vi "mfTxTrchCoder.vi"(7 "coder_type":dbl, 8 "error in (no error)":errorcluster caption="错误输入（无错误）", 9 "input_num":dbl, 10 "pdch_data":dbl[](array[numeric]), 11 "Path":path) -> (0 "error out":errorcluster caption="错误输出", 3 "out_data":dbl[](array[numeric]))   [LabVIEW 2015]
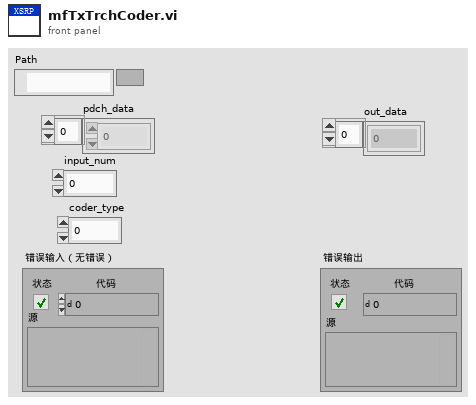
[diagram p1: front panel]
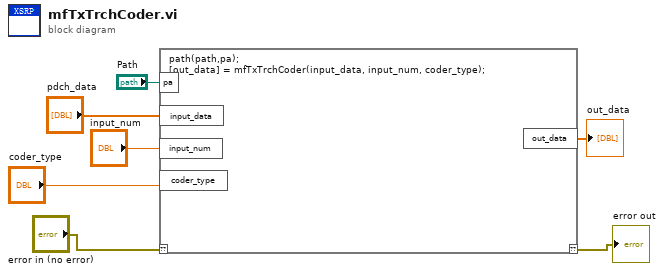
[diagram p0: block diagram]
diagram:
  n1 = script code="path(path,pa);\n[out_data] = mfTxTrchCoder(input_data, input_num, coder_type);"("??"="error in (no error)", "pa"="Path", "input_data"="pdch_data", "input_num"="input_num", "coder_type"="coder_type") -> ("??"=→"error out":errorcluster, "out_data"=→"out_data":dbl[])
